vi "DiffDriveGlobals.vi"() -> ()   [LabVIEW 2025]
panel:
  out "Right Motor Init":bool
  out "Left Motor Init":bool
  out "RightMotorOutput":dbl
  out "LeftMotorOutput":dbl
  out "RightSpeedTargetFtSec":dbl
  out "LeftSpeedTargetFtSec":dbl
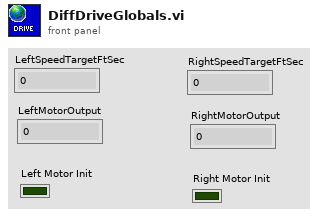
[diagram p1: front panel]
diagram:
